vi "endEventToString.vi"(8 "error in (no error)":errorcluster, 11 "RampToneDown in":refnum<class "RampToneDown.lvclass">) -> (0 "error out":errorcluster, 3 "RampToneDown out":refnum<class "RampToneDown.lvclass">)   [LabVIEW 2009, in "Tools.lvlib" / "Scripting.lvlib" / "RampToneDown.lvclass"]
uses:
  RampToneDown.lvclass
  RampTone/RampTone.lvclass
panel:
  out "eventStringArray":string[](array[string])
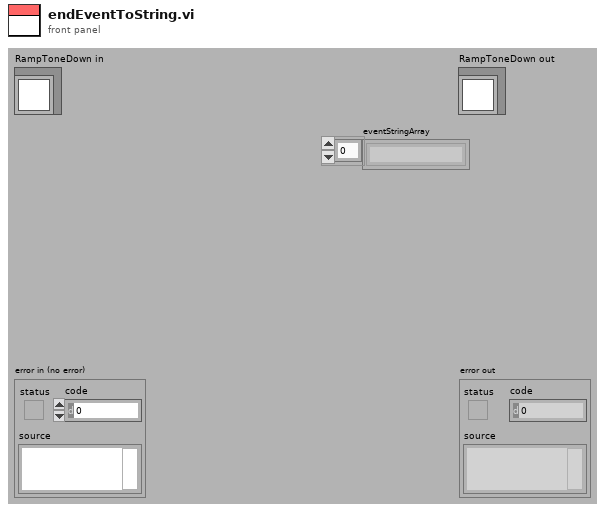
[diagram p1: front panel]
types:
  T1 = cluster{"rampTime":dbl, "timeStep":dbl, "dataValueStep":dbl}
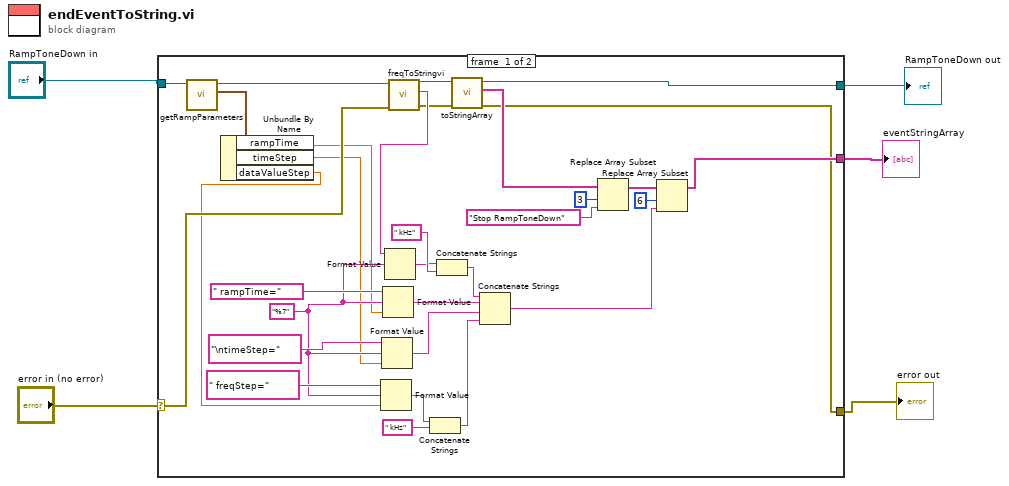
[diagram p0: block diagram]
diagram:
  n1 = case shown="No Error" "error in (no error)" {
    selector: "error in (no error)" -> [w17 w37]
    tunnel: [w6 w37] -> w2
    tunnel: [w23 _] -> w1
    tunnel: "RampToneDown in" -> [w16 w38]
    tunnel: [w7 w38] -> w5
    frame #0 {
      w22 = "%7"
      n2 = call "getRampParameters.vi"("RampTone in"=w16) -> ("RampParameters"=w14:T1, "RampTone out"=w15:refnum<class "RampToneDown.lvclass">)  [unwired: 8 in, 1 out]
      n3 = Unbundle By Name(w14) -> ("rampTime"=w13:dbl, "timeStep"=w12:dbl, "dataValueStep"=w11:dbl)
      n4 = Format Value(string ("")=" freqStep=", format string=w22, value (0)=w11) -> (output string=w26:string)
      n5 = Format Value(string ("")="\ntimeStep=", format string=w22, value (0)=w12) -> (output string=w28:string)
      n6 = Format Value(string ("")=" rampTime=", format string=w22, value (0)=w13) -> (output string=w29:string)
      n7 = call-dynamic "freqToStringvi.vi"("error in (no error)"=w17, "SingleTone in"=w15) -> ("error out"=w9:errorcluster, "frequency"=w18:string, "SingleTone out"=w10:refnum<class "RampToneDown.lvclass">)  [unwired: 7 in]
      n8 = Format Value(string ("")=w18, format string=w22) -> (output string=w20:string)  [unwired: 1 in]
      n9 = Concatenate Strings(w26, " kHz") -> (w24:string)
      n10 = Concatenate Strings(w20, " kHz") -> (w19:string)
      n11 = call-dynamic "toStringArray.vi"("error in (no error)"=w9, "RampToneDown in"=w10) -> ("error out"=w6:errorcluster, "eventStringArray"=w8:string[], "RampToneDown out"=w7:refnum<class "RampToneDown.lvclass">)  [unwired: 7 in]
      n12 = Concatenate Strings(w19, w29, w28, w24) -> (w27:string)
      n13 = Replace Array Subset(array=w8, new element="Stop RampToneDown", index=3) -> (w32:string[])
      n14 = Replace Array Subset(array=w32, new element=w27, index=6) -> (w23:string[])
    }
    frame #1 {
    }
  }
  "error out" <- w2
  "RampToneDown out" <- w5
  "eventStringArray" <- w1
